vi "9093_第5回目課題_山口修平.vi"() -> ()   [LabVIEW 2020]
uses:
  <vilib>/Utility/file.llb/Write Delimited Spreadsheet (DBL).vi
panel:
  out "出力":dbl
  in  "Path":path
  out "波形チャート":dbl(graph)
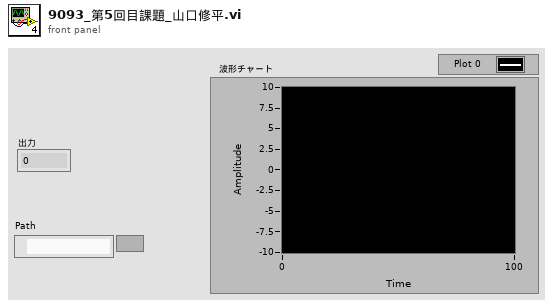
[diagram p1: front panel]
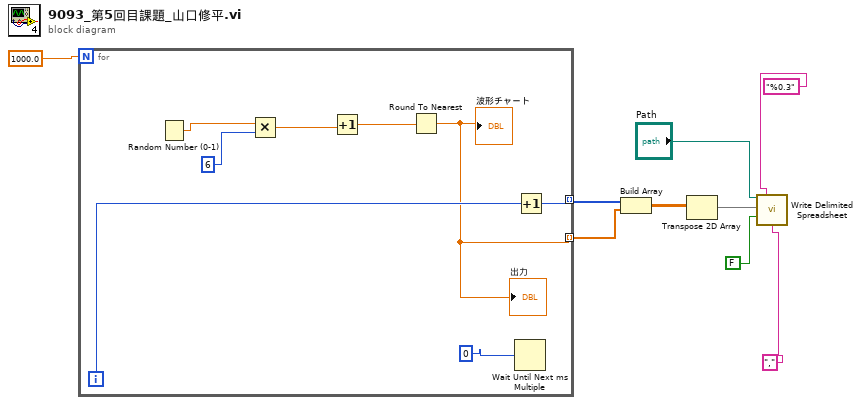
[diagram p0: block diagram]
diagram:
  n1 = for {
    N: 1000.0 -> [_]
    tunnel: [w12] -> w7 mode=indexing
    tunnel: [w10] -> w8 mode=indexing
    i -> [w11]
    n2 = Random Number (0-1)() -> (number: 0 to 1=w17:dbl)
    n3 = Multiply(x=w17, y=6) -> (x*y=w16:dbl)
    n4 = Increment(x=w16) -> (x+1=w15:dbl)
    n5 = Round To Nearest(number=w15) -> (nearest integer value=w10:dbl)
    "波形チャート" <- w10
    "出力" <- w10
    n6 = Wait Until Next ms Multiple(millisecond multiple=0) -> ()  [unwired: 1 out]
    n7 = Increment(x=w11) -> (x+1=w12:i32)
  }
  n8 = Build Array(w7, w8) -> (w6:dbl[][])
  n9 = Transpose 2D Array(2D array=w6) -> (transposed array=w5:dbl[][])
  n10 = call-poly <vilib>:"Write Delimited Spreadsheet.vi"("file path (dialog if empty)"="Path", "format (%.3f)"="%0.3", "2D data"=w5, "append to file? (new file:F)"=FALSE, "delimiter (\\t)"=",") -> ()  [unwired: 9 in, 2 out]
